vi "Test Glyph on Method Not Started Correct on Start Selective.vi"(8 "error in (no error)":errorcluster, 11 "Result Model Tests in":refnum<class "Result Model Test Enumeration.lvclass">) -> (0 "error out":errorcluster, 3 "Result Model Tests out":refnum<class "Result Model Test Enumeration.lvclass">)   [LabVIEW 2020, in "Result Model Test Enumeration.lvclass"]
uses:
  Result Model Test Enumeration.lvclass
  C:/Program Files (x86)/National Instruments/LabVIEW 2020/vi.lib/Astemes/LUnit/Test Case.lvclass
  <vilib>/Astemes/LUnit/Test Case.lvclass/Test Case.ctl
  206db1ee-aa99-40b9-8881-171f2a77c34b.vi
  <vilib>/Astemes/LUnit/Palette/Pass.vi
  <vilib>/Astemes/LUnit/Palette/Fail.vi
  <vilib>/Astemes/LUnit/Compare Variants.vi
  <vilib>/Astemes/LUnit/Describe Comparison.vi
  <vilib>/Astemes/LUnit/Set Assertion Type.vi
  <vilib>/Astemes/LUnit/Add test result.vi
  <vilib>/Astemes/LUnit/Variant to string.vi
  <vilib>/Astemes/LUnit/LUnit Record Assertion Result.vi
  <vilib>/Astemes/LUnit/LUnit Aggregate Assertion Results.vi
  <vilib>/Astemes/LUnit/Method Result/LUnit Merge Status.vi
  <vilib>/Astemes/LUnit/LUnit Concatenate result strings.vi
  <vilib>/Utility/Data Type/Get Type Information.vi
  <vilib>/Utility/LVClass/Get LV Class Name.vi
  Result Model Test Enumeration.lvclass/Result Model Test Enumeration.ctl
  Result Model/Result Model.lvclass
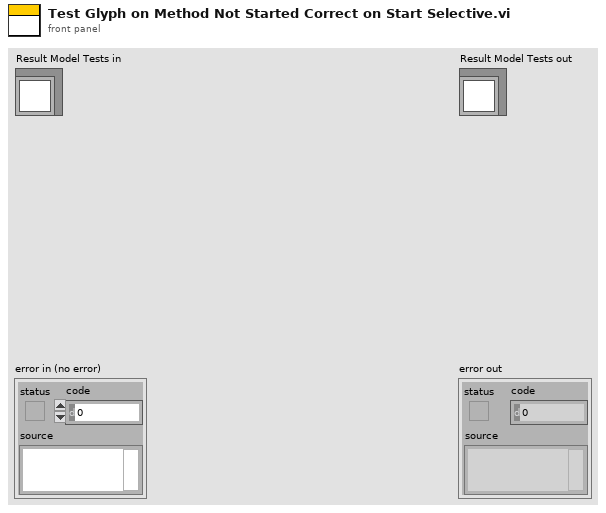
[diagram p1: front panel]
types:
  T1 = cluster{"Left Cell String":string, "Child Text":string[], "Child Tag":string, "Item Indent":i32, "Child Only?":bool, "Glyph Index":i32}[]
  T2 = cluster{"Left Cell String":string, "Child Text":string[], "Child Tag":string, "Item Indent":i32, "Child Only?":bool, "Glyph Index":i32}
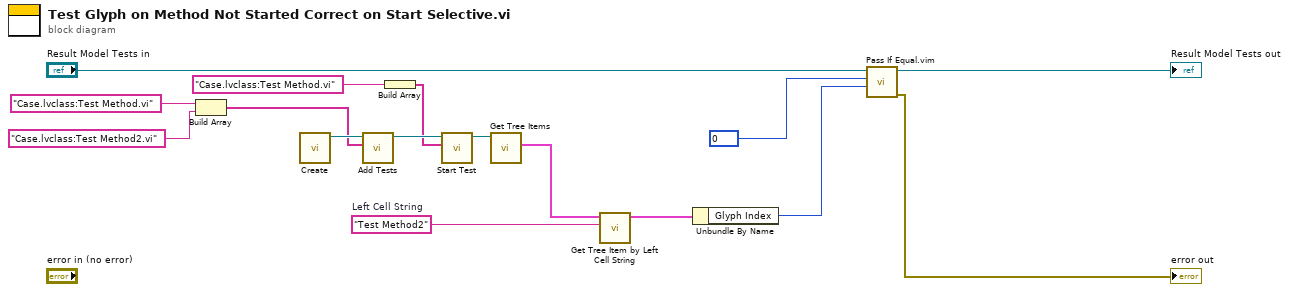
[diagram p0: block diagram]
diagram:
  w7 = "Test Method2"  # Left Cell String
  n1 = Build Array("Case.lvclass:Test Method.vi" ("String"), "Case.lvclass:Test Method2.vi" ("String")) -> (w10:string[])
  n2 = call "Create.vi"() -> ("Result Model out"=w15:refnum<class "Result Model.lvclass">)  [unwired: 11 in]
  n3 = call "Add Tests.vi"("Tests"=w10, "Result Model In"=w15) -> ("Result Model Out"=w5:refnum<class "Result Model.lvclass">)  [unwired: 9 in]
  n4 = Build Array("Case.lvclass:Test Method.vi" ("String")) -> (w1:string[])
  n5 = call "Start Test.vi"("Tests"=w1, "Result Model In"=w5) -> ("Result Model Out"=w4:refnum<class "Result Model.lvclass">)  [unwired: 9 in]
  n6 = call "Get Tree Items.vi"("Result Model In"=w4) -> ("Tree Items"=w14:T1)  [unwired: 10 in]
  n7 = call "Get Tree Item by Left Cell String.vi"("Left Cell String"=w7, "Tree Items"=w14) -> ("Item"=w12:T2)  [unwired: 9 in]
  n8 = Unbundle By Name(w12) -> ("Glyph Index"=w11:i32)
  n9 = call "Pass If Equal.vim"("Actual"=w11, "Expected"=0 ("Listbox Symbol Ring Constant"), "LUnit Test Case In"="Result Model Tests in") -> ("error out"=→"error out":errorcluster, "LUnit Test Case Out"=→"Result Model Tests out":refnum<class "Result Model Test Enumeration.lvclass">)  [unwired: 7 in]
